vi "Resample N Pairs of Arrays (single shot).vi"(0 "Multiple XY-data in":cluster{"X-array":dbl[], "Y-array":dbl[]}[](array[cluster]) {"Y-array" format="%.2p"; "X-array" format="%.2p"}, 5 "dt":dbl=1.0 format="%.2p", 7 "t0":dbl=-inf format="%.2p", 9 "interpolation mode":u16(ring)=1 items=["coerce", "linear", "spline", "FIR filter"], 11 "error in (no error)":errorcluster) -> (4 "resampled waveforms out":waveform(dbl)[](array[waveform]), 6 "Multiple XY-data out":cluster{"X-array":dbl[], "Y-array":dbl[]}[](array[cluster]) {"Y-array" format="%.2p"; "X-array" format="%.2p"}, 10 "used t0's":dbl[](array[numeric]) format="%.2p", 14 "t0 adjusted warnings":bool[](array[boolean]), 15 "error out":errorcluster)   [LabVIEW 2020, in "NI_MAPro.lvlib"]
doc: "Resamples input waveforms or data according to the user-defined <B>t0</B> and <B>dt</B> values.\n\nWire data to the waveform or data input to determine the polymorphic instance to use or manually select the instance."
uses:
  NI_MAPro.lvlib
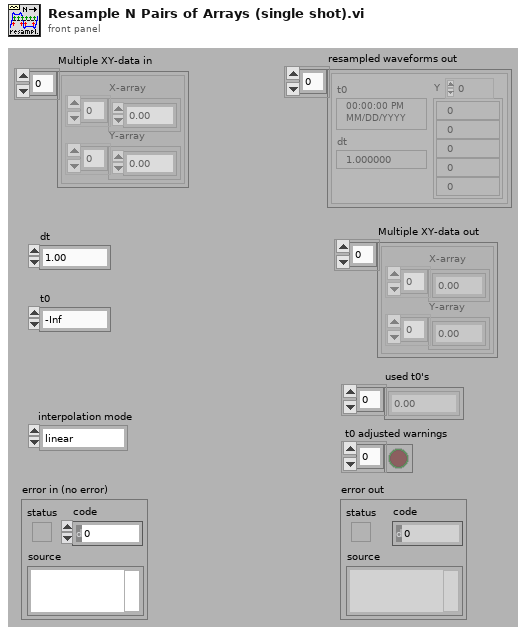
[diagram p1: front panel]
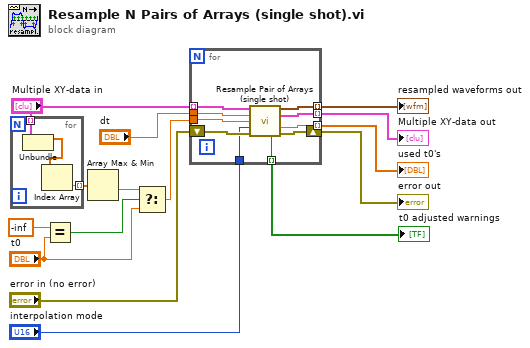
[diagram p0: block diagram]
diagram:
  n1 = for {
    tunnel: [w16] -> w8 mode=indexing
    tunnel: "Multiple XY-data in" -> [w18] mode=indexing
    n2 = Unbundle(w18) -> ("X-array"=w17:dbl[])  [unwired: 1 out]
    n3 = Index Array(array=w17) -> (element=w16:dbl)  [unwired: 1 in]
  }
  n4 = Equal?(x=-inf, y="t0") -> (x = y?=w3:bool)
  n5 = Array Max & Min(array=w8) -> (min value=w6:dbl)  [unwired: 3 out]
  n6 = Select(t=w6, s=w3, f="t0") -> (s? t:f=w7:dbl)
  n7 = for {
    tunnel: "Multiple XY-data in" -> [w20] mode=indexing
    shift-right: [w27] -> w14
    shift-left: "error in (no error)" -> [w28]
    tunnel: [w26] -> w13 mode=indexing
    tunnel: [w25] -> w12 mode=indexing
    tunnel: [w24] -> w11 mode=indexing
    tunnel: "dt" -> [w23]
    tunnel: w7 -> [w22]
    tunnel: "interpolation mode" -> [w21]
    tunnel: [w19] -> w1 mode=indexing
    n8 = call "Resample Pair of Arrays (single shot).vi"("XY-data in"=w20, "dt"=w23, "t0"=w22, "interpolation mode"=w21, "error in (no error)"=w28) -> ("resampled waveform out"=w25:waveform(dbl), "XY-data out"=w19:cluster{"X-array":dbl[], "Y-array":dbl[]}, "used t0"=w26:dbl, "t0 adjusted warning"=w24:bool, "error out"=w27:errorcluster)  [unwired: 6 in]
  }
  "error out" <- w14
  "resampled waveforms out" <- w12
  "used t0's" <- w13
  "t0 adjusted warnings" <- w11
  "Multiple XY-data out" <- w1
